vi "Hood Control.vi"(7 "Vision":bool, 8 "Top":T1, 11 "Bottom":T1) -> (0 "HoodSpeed":dbl, 1 "Voltage":dbl, 2 "Shoter Angle":dbl)   [LabVIEW 2011]
uses:
  <vilib>/Rock Robotics/WPI/DigitalInput/WPI_DigitalInputDevRef.ctl
  <vilib>/Rock Robotics/SystemInterfaces/DIO/FPGA_DIOChannel.ctl
  <vilib>/Rock Robotics/SystemInterfaces/Typedef/FPGA_TypedefDigitalModule.ctl
  <vilib>/Rock Robotics/WPI/AnalogChannel/WPI_AnalogChannelDevRef.ctl
  <vilib>/Rock Robotics/SystemInterfaces/Typedef/FPGA_TypedefAnalogModule.ctl
  <vilib>/Rock Robotics/SystemInterfaces/AI/FPGA_AIChannel.ctl
  System Set Points and States.vi
  Robot Global Data.vi
panel:
  out "Target Info[0].Distance (ft)":dbl
  in  "AIDeviceRef":T4
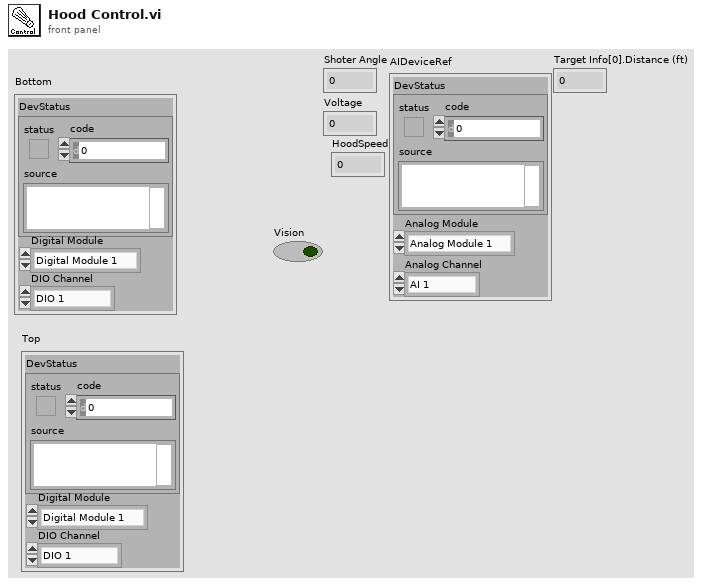
[diagram p1: front panel]
types:
  T1 = typedef "WPI_DigitalInputDevRef.ctl" = cluster{"DevStatus":errorcluster, "DIO Channel":T2, "Digital Module":T3}
  T2 = typedef "FPGA_DIOChannel.ctl" = enum8{"DIO 1", "DIO 2", "DIO 3", "DIO 4", "DIO 5", "DIO 6", "DIO 7", "DIO 8", "DIO 9", "DIO 10", "DIO 11", "DIO 12", "DIO 13", "DIO 14", "Invalid"}
  T3 = typedef "FPGA_TypedefDigitalModule.ctl" = enum16{"Digital Module 1", "Digital Module 2"}
  T4 = typedef "WPI_AnalogChannelDevRef.ctl" = cluster{"DevStatus":errorcluster, "Analog Module":T5, "Analog Channel":T6}
  T5 = typedef "FPGA_TypedefAnalogModule.ctl" = enum16{"Analog Module 1", "Analog Module 2"}
  T6 = typedef "FPGA_AIChannel.ctl" = enum8{"AI 1", "AI 2", "AI 3", "AI 4", "AI 5", "AI 6", "AI 7", "AI 8", "Invalid"}
  T7 = cluster{"Position":cluster{"X":dbl, "Y":dbl}, "Distance (ft)":dbl}[]
  T8 = cluster{"Target Info[0]":cluster{"Position":cluster{"X":dbl, "Y":dbl}, "Distance (ft)":dbl}, "Target Info[1]":cluster{"Position":cluster{"X":dbl, "Y":dbl}, "Distance (ft)":dbl}, "Target Info[2]":cluster{"Position":cluster{"X":dbl, "Y":dbl}, "Distance (ft)":dbl}, "Target Info[3]":cluster{"Position":cluster{"X":dbl, "Y":dbl}, "Distance (ft)":dbl}, "Target Info[4]":cluster{"Position":cluster{"X":dbl, "Y":dbl}, "Distance (ft)":dbl}, "Target Info[5]":cluster{"Position":cluster{"X":dbl, "Y":dbl}, "Distance (ft)":dbl}, "Target Info[6]":cluster{"Position":cluster{"X":dbl, "Y":dbl}, "Distance (ft)":dbl}, "Target Info[7]":cluster{"Position":cluster{"X":dbl, "Y":dbl}, "Distance (ft)":dbl}, "Target Info[8]":cluster{"Position":cluster{"X":dbl, "Y":dbl}, "Distance (ft)":dbl}}
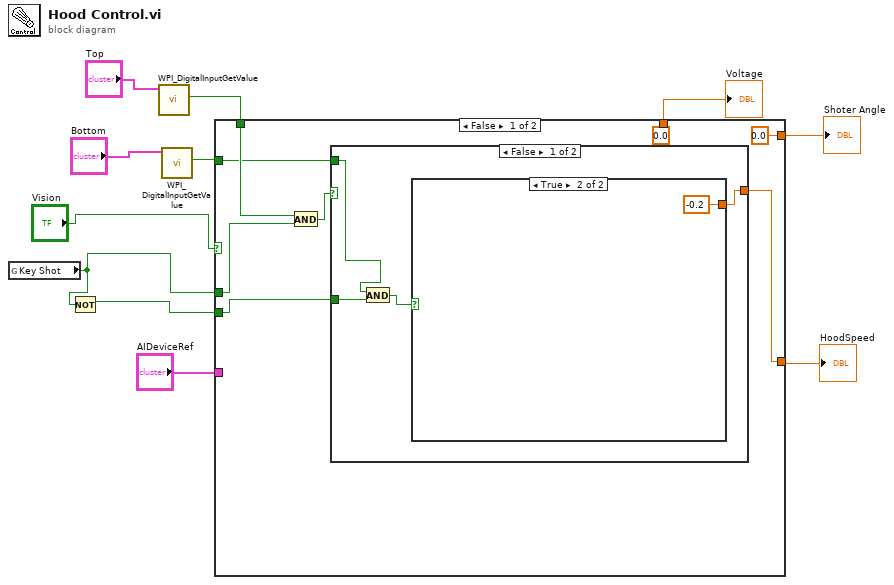
[diagram p0: block diagram]
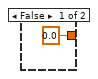
[diagram p2: hidden frame]
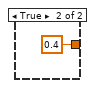
[diagram p3: hidden frame]
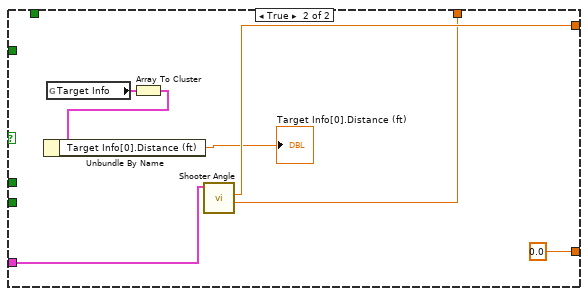
[diagram p4: hidden frame]
diagram:
  n1 = global read "System Set Points and States.vi" "Key Shot"() -> (w2:bool)
  n2 = Not(x=w2) -> (.not. x?=w1:bool)
  n3 = call <vilib>:"WPI_DigitalInputGetValue.vi"("DigitalInputDevRef"="Top") -> ("Value"=w3:bool)  [unwired: 8 in, 2 out]
  n4 = call <vilib>:"WPI_DigitalInputGetValue.vi"("DigitalInputDevRef"="Bottom") -> ("Value"=w8:bool)  [unwired: 8 in, 2 out]
  n5 = case shown="False" "Vision" {
    tunnel: w1 -> [w15 _]
    tunnel: w2 -> [w19 _]
    tunnel: [w16 0.0 ("Output")] -> w10
    tunnel: w8 -> [w14 _]
    tunnel: [0.0 ("Shoter Angle") w33] -> w7
    tunnel: [0.0 ("Voltage") w32] -> w6
    tunnel: "AIDeviceRef" -> [_ w31]
    tunnel: w3 -> [w18 _]
    frame False {
      n6 = And(x=w18, y=w19) -> (x .and. y?=w17:bool)
      n7 = case shown="False" w17 {
        tunnel: [w21 0.4 ("Voltage")] -> w16
        tunnel: w15 -> [w23 _]
        tunnel: w14 -> [w20 _]
        frame False {
          n8 = And(x=w20, y=w23) -> (x .and. y?=w22:bool)
          n9 = case shown="True" w22 {
            tunnel: [0.0 ("Voltage") -0.2 ("Voltage")] -> w21
            frame False {
            }
            frame True {
            }
          }
        }
        frame True {
        }
      }
    }
    frame True {
      n10 = global read "Robot Global Data.vi" "Target Info"() -> (w30:T7)
      n11 = Array To Cluster(array=w30) -> (cluster=w29:T8)
      n12 = Unbundle By Name(w29) -> ("Target Info[0].Distance (ft)"=→"Target Info[0].Distance (ft)":dbl)
      n13 = call "Shooter Angle.vi"("AIDeviceRef"=w31) -> ("Voltage"=w32:dbl, "Shoter Angle"=w33:dbl)  [unwired: 9 in]
    }
  }
  "Shoter Angle" <- w7
  "Voltage" <- w6
  "HoodSpeed" <- w10
